vi "readProgramStats.vi"(8 "error in (no error)":errorcluster, 11 "ILC in":refnum<class "ILC.lvclass">) -> (0 "error out":errorcluster, 2 "Response":string, 3 "ILC out":refnum<class "ILC.lvclass">)   [LabVIEW 2015, in "ILCCommon.lvlib" / "ILC.lvclass"]
uses:
  <userlib>/Common/ILC/ILC/ILC.lvclass
  <userlib>/Common/ILC/ILC/ILC.lvclass/ILC.ctl
  <userlib>/Common/SerialProtocols/SerialCommunicator/SerialCommunicator.lvclass
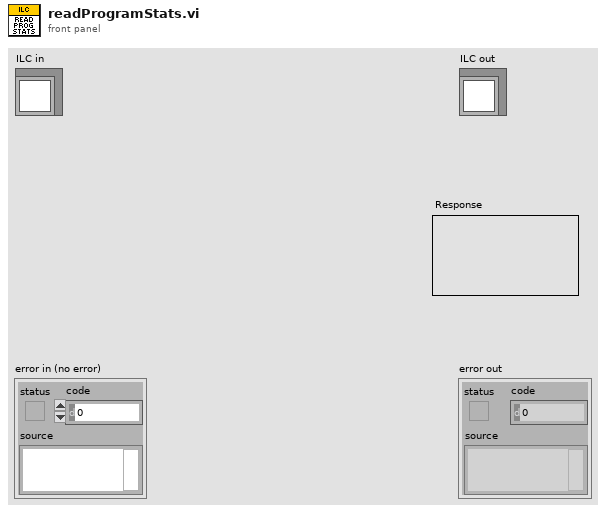
[diagram p1: front panel]
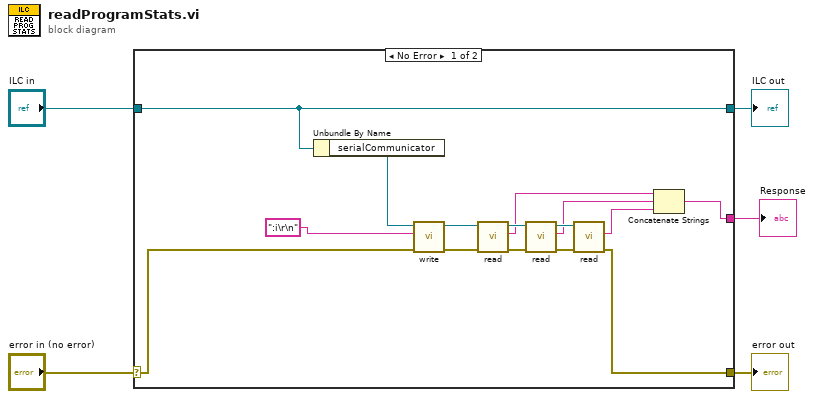
[diagram p0: block diagram]
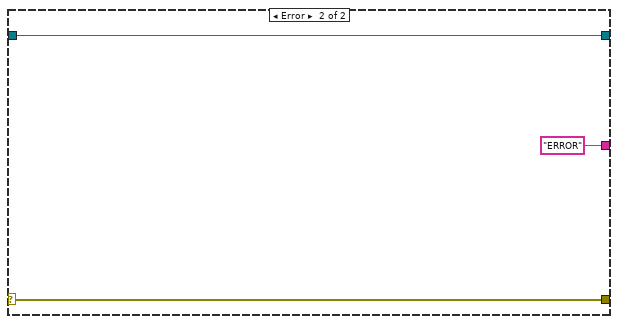
[diagram p2: hidden frame]
diagram:
  n1 = case shown="No Error" "error in (no error)" {
    selector: "error in (no error)" -> [w17 w23]
    tunnel: [w6 w23] -> w4
    tunnel: [w20 w22] -> w2
    tunnel: "ILC in" -> [w20 w22]
    tunnel: [w7 "ERROR" ("stringRead")] -> w1
    frame No Error {
      n2 = Unbundle By Name(w20) -> ("serialCommunicator"=w18:refnum<class "SerialCommunicator.lvclass">)
      n3 = call-dynamic "write.vi"("error in (no error)"=w17, "writeString"=":i\r\n", "SerialCommunicator in"=w18) -> ("error out"=w16:errorcluster, "SerialCommunicator out"=w15:refnum<class "SerialCommunicator.lvclass">)  [unwired: 7 in]
      n4 = call-dynamic "read.vi"("error in (no error)"=w16, "SerialCommunicator in"=w15) -> ("error out"=w14:errorcluster, "stringRead"=w10:string, "SerialCommunicator out"=w13:refnum<class "SerialCommunicator.lvclass">)  [unwired: 7 in]
      n5 = call-dynamic "read.vi"("error in (no error)"=w14, "SerialCommunicator in"=w13) -> ("error out"=w12:errorcluster, "stringRead"=w9:string, "SerialCommunicator out"=w11:refnum<class "SerialCommunicator.lvclass">)  [unwired: 7 in]
      n6 = call-dynamic "read.vi"("error in (no error)"=w12, "SerialCommunicator in"=w11) -> ("error out"=w6:errorcluster, "stringRead"=w8:string)  [unwired: 7 in, 1 out]
      n7 = Concatenate Strings(w10, w9, w8) -> (w7:string)
    }
    frame Error {
    }
  }
  "error out" <- w4
  "ILC out" <- w2
  "Response" <- w1
